vi "PatchMultipartMethod.vi"(6 "Headers":cluster{"Name":string, "Value":string}[](array[cluster]), 8 "error in (no error)":errorcluster, 9 "Multpart/Form-Data":T1(array[cluster]), 10 "Endpoint URL":string, 11 "Request in":refnum<class "Request.lvclass">) -> (0 "error out":errorcluster, 2 "Response out":refnum<class "Response.lvclass">, 3 "Request out":refnum<class "Request.lvclass">)   [LabVIEW 2016]
uses:
  Request.lvclass
  Response.lvclass
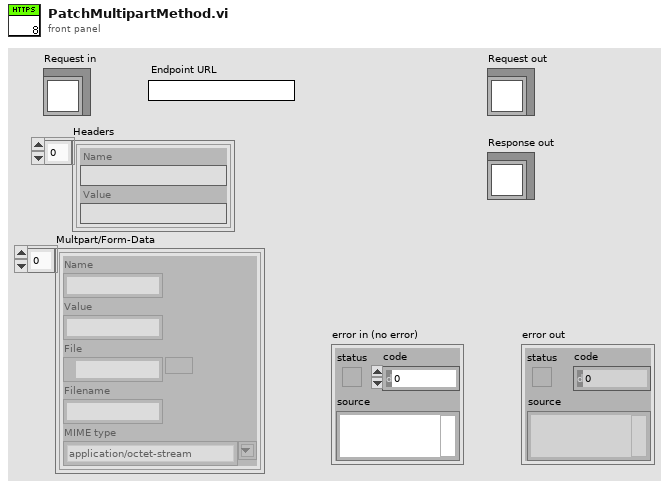
[diagram p1: front panel]
types:
  T1 = cluster{"Name":string, "Value":string, "File":path, "Filename":string, "MIME type":string}[]
  T2 = enum16{"PATCH_MULTIPART", "POST_MULTIPART", "PATCH", "DELETE", "HEAD", "PUT", "GET"}
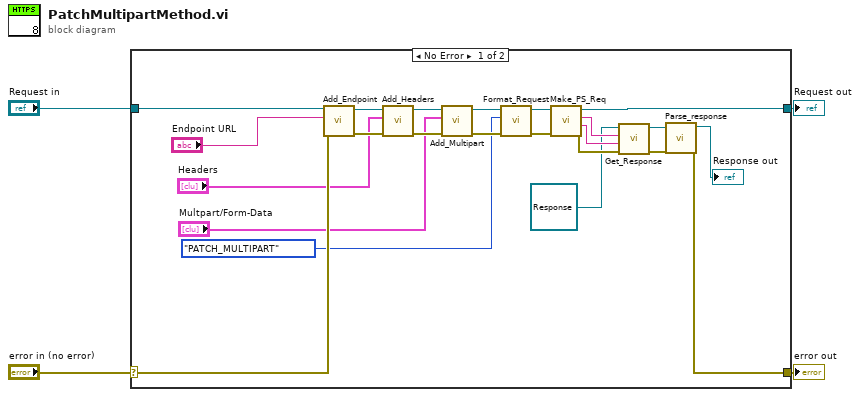
[diagram p0: block diagram]
diagram:
  n1 = case shown="No Error" "error in (no error)" {
    selector: "error in (no error)" -> [w11 w29]
    tunnel: [w10 w29] -> w3
    tunnel: [w21 w28] -> w1
    tunnel: "Request in" -> [w24 w28]
    frame No Error {
      n2 = call "Add_Endpoint.vi"("error in (no error)"=w11, "Endpoint URL"="Endpoint URL", "Request in"=w24) -> ("error out"=w12:errorcluster, "Request out"=w27:refnum<class "Request.lvclass">)  [unwired: 7 in]
      n3 = call "Add_Headers.vi"("error in (no error)"=w12, "Headers"="Headers", "Request in"=w27) -> ("error out"=w13:errorcluster, "Request out"=w26:refnum<class "Request.lvclass">)  [unwired: 7 in]
      n4 = call "Add_Multipart.vi"("error in (no error)"=w13, "Multpart/Form-Data"="Multpart/Form-Data", "Request in"=w26) -> ("error out"=w14:errorcluster, "Request out"=w25:refnum<class "Request.lvclass">)  [unwired: 7 in]
      n5 = call "Format_Request.vi"("error in (no error)"=w14, "Request"=T2."PATCH_MULTIPART", "Request in"=w25) -> ("error out"=w15:errorcluster, "Request out"=w22:refnum<class "Request.lvclass">)  [unwired: 7 in]
      n6 = call "Make_PS_Req.vi"("error in (no error)"=w15, "Request in"=w22) -> ("error out"=w16:errorcluster, "standard error"=w19:string, "standard output"=w20:string, "Request out"=w21:refnum<class "Request.lvclass">)  [unwired: 6 in]
      n7 = call "Get_Response.vi"("error in (no error)"=w16, "PS Error"=w19, "PS Response"=w20, "Response in"=refnum<class "Response.lvclass"> refnum) -> ("error out"=w17:errorcluster, "Response out"=w18:refnum<class "Response.lvclass">)  [unwired: 6 in]
      n8 = call "Parse_response.vi"("error in (no error)"=w17, "Response in"=w18) -> ("error out"=w10:errorcluster, "Response out"=→"Response out":refnum<class "Response.lvclass">)  [unwired: 8 in]
    }
    frame Error {
    }
  }
  "error out" <- w3
  "Request out" <- w1
